vi "SVT FFT Spectrum Subset (Mag-Phase).vi"   [LabVIEW 2017]
doc: "Computes a subset of the FFT spectrum of <B>scaled signal [EU]</B>. The subset is defined by <B>frequency range</B>. FFT results are returned as <B>magnitude [dB EU]</B> and <B>phase [degrees]</B>. Each block of data corresponds to a single FFT block and has to be passed individually to this VI. You can use this polymorphic VI to analyze signals from a single channel or from N channels. The data type you wire to the <B>scaled signal [EU]</B> input determines the polymorphic instance to use."
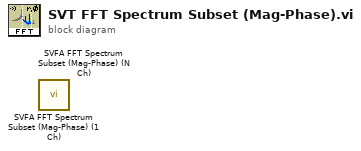
[diagram p0: block diagram]
diagram:
  n1 = call <vilib>:"SVFA FFT Spectrum Subset (Mag-Phase) (1 Ch).vi"() -> ()  [unwired: 12 in, 8 out]
  n2 = call <vilib>:"SVFA FFT Spectrum Subset (Mag-Phase) (N Ch).vi"() -> ()  [unwired: 12 in, 8 out]
